vi "Test.vi"() -> ()   [LabVIEW 2010]
uses:
  <vilib>/DAQmx/read.llb/DAQmx Read.vi
  <vilib>/DAQmx/read.llb/DAQmx Read (Analog 2D DBL NChan NSamp).vi
  Create Dataset 2D Double.vi
  <vilib>/daqmx/miscellaneous.llb/DAQmx Fill In Error Info.vi
  Append To Dataset 2D Double.vi
  HDF5Tools.lvlib
panel:
  out "output array":dbl[](array[numeric])
  out "data 2":dbl[][](array[numeric]) format="%0.2f"
  out "size(s)":i32[](array[numeric])
  out "data":dbl[][](graph)
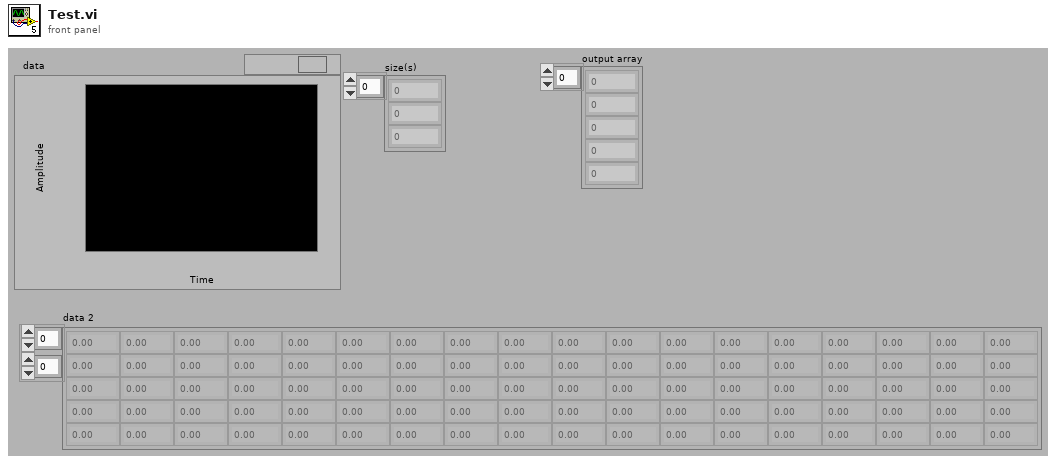
[diagram p1: front panel]
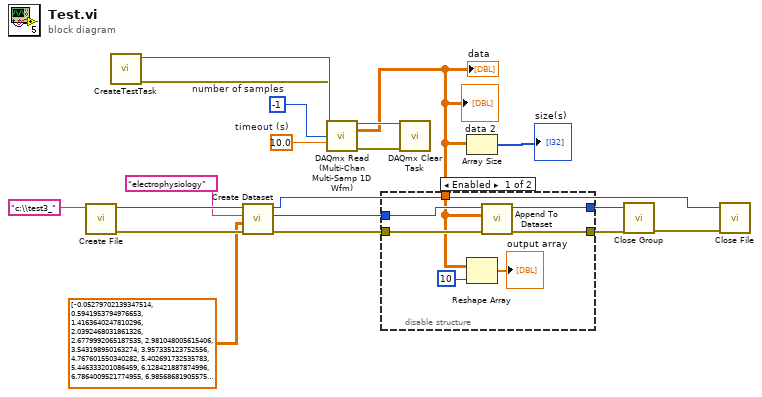
[diagram p0: block diagram]
diagram:
  w18 = 10.0  # timeout (s)
  w19 = -1  # number of samples
  n1 = call "Create File.vi"("File name"="c:\\test3_") -> ("Error out"=w9:errorcluster, "file_id"=w11:i32)  [unwired: 8 in]
  n2 = call "CreateTestTask.vi"() -> ("error out"=w14:errorcluster, "task out"=w15:refnum<k21>)  [unwired: 10 in]
  n3 = call-poly "Create Dataset.vi"("error in (no error)"=w9, "Data type"=dbl[][] [[-0.05279702139347514, 0.5941953794976653, 1.4163640247810296, 2.0392468031861326, 2.6779992065187535, 2.981048005615406, 3.543198950163274, 3.957335123752556, 4.767601550340282, 5.402691732535783, 5.446333201086459, 6.128421887874996, 6.7864009521774955, 6.985686819055758, 7.252723776970733, 7.696157719656972, 8.288827173680838, 8.26258125553148, 9.01364177373577, 8.951078829309976, 9.093600268562883, 9.45158238471633, 9.587694936979277, 9.609973448896756, 9.969481490524004, 9.938657795953246, 9.722586748863186, 9.497054963835566, 9.711600085451826, 9.554734946745201, 9.12961210974456, 9.220862453077793, 8.817712942899869, 8.655354472487563, 8.361461226233711, 7.8505813776055176, 7.7626880703146455, 6.990874965666677, 6.484572893459884, 5.98620563371685, 5.8729819635609, 4.979094821008942, 4.751731925412763, 4.029969176305429, 3.794366283150731, 3.174535355693228, 2.468947416608173, 1.6562395092623676, 1.1597033600878932, 0.5365153965880306, 0.06256294442579424, -0.32349620044557026, -0.9436323129978332, -1.9043549913022249, -2.652668843653676, -2.8943754387035736, -3.507797479171117, -3.9820551164281137, -4.6092104861598555, -5.171971800897244, -5.940122684408093, -6.327707754753257, -6.4226203192236095, -7.336954863124485, -7.196264534440138, -7.905209509567553, -7.9229102450636315, -8.770104068117313, -8.714255195776238, -8.944364757225257, -9.288308359019746, -9.182714316232795, -9.546189764091922, -9.67223120822779, -9.77782525101474, -9.749137852107303, -9.88952299569689, -9.640186773277993, -9.45890682699057, -9.431440168462172, -9.213538010803552, -8.856166264839626, -8.534501174962616, -8.512527848139896, -7.985168004394666, -7.706228827784051, -7.265541550950651, -7.314065981017487, -6.391796624652852, -6.2779625843073825, -5.897701956236458, -4.919278542435987, -4.865260780663473, -4.280831324198126, -3.3771782586138492, -3.293252357554857, -2.196722312082278, -1.564989165929136, -1.4697714163640248, -0.5999938962981048], [1.0998870815149389, 1.391338847010712, 2.226325266273995, 2.531510361033967, 3.3530686361278117, 3.595080416272469, 4.5603808709982605, 5.070039979247413, 5.275124362926115, 5.736564226203193, 6.082033753471481, 6.618549150059511, 7.011322367015595, 7.806329538865322, 7.701345866267891, 8.356578264717552, 8.833582567827387, 8.666646320993683, 8.846095156712547, 9.324320200201422, 9.720450453199867, 9.432355723746452, 9.642323068941312, 9.807123020111698, 9.539475692007203, 9.652699362163151, 9.492477187414167, 9.311807611316263, 9.423200170903653, 8.887295144505142, 8.654744102298043, 8.744163335062716, 8.549150059511094, 8.281197546311837, 7.417828913235877, 7.181920834986419, 6.910000915555284, 6.73818170720542, 5.87176122318186, 5.248878444776757, 5.085299233985412, 4.293954283272805, 3.6783959471419414, 3.083590197454756, 2.8113650929288614, 2.481460005493332, 1.6397595141453292, 0.7055879390850551, 0.5490279854731895, -0.10071108127079073, -0.9332560197759942, -1.6165654469435713, -1.9507431257057406, -2.621845149082919, -3.4580523087252417, -3.598437452314829, -4.082155827509385, -4.654683065279092, -5.513168736838892, -5.7777642139957885, -6.416821802423169, -7.009186071352275, -7.072969756157109, -7.345805230872524, -7.9396954252754295, -8.36634418774987, -8.741416669209876, -8.781395916623431, -9.282509842219307, -9.110385448774682, -9.584948271126438, -9.68230231635487, -9.35300759910886, -9.761345255897702, -9.761345255897702, -9.597460860011598, -9.765923032319101, -9.403057954649494, -9.547410504470962, -8.852198858607746, -9.069795831171605, -8.908658101138341, -8.37000640888699, -8.174382763145848, -7.771843623157445, -7.565843684194464, -6.823633533738212, -6.516006958220161, -6.160771507919553, -5.698416089358195, -5.094759971922971, -4.2780846583452865, -3.9252906888027588, -3.087252418591876, -2.5794244209112827, -2.325510422070986, -1.573839533677175, -0.9857478560747093, -0.5029450361644338, 0.195623645741142], [1.7447431867427594, 2.551347392193365, 3.0491042817468794, 3.7076937162388988, 3.783379619739372, 4.2695394756920075, 4.863734855189673, 5.7695242164372695, 6.2462233344523455, 6.539506210516678, 6.890774254585406, 7.264931180761131, 7.50144962920011, 7.911313211462752, 8.242744224372082, 8.625751518295846, 9.227271340067752, 9.216589861751151, 9.583422345652638, 9.604480117191077, 9.89410077211829, 9.45005645924253, 9.611499374370556, 9.957274086733603, 9.646900845362712, 9.44792016357921, 9.33622241889706, 9.519333475753044, 9.179357280190436, 8.966032898953214, 8.554948576311533, 8.285470137638479, 8.010193182164983, 7.353740043336283, 7.1254615924558244, 6.478469191564684, 6.355479598376415, 6.026184881130406, 5.041352580339976, 4.622943815424055, 4.001892147587512, 3.7336344492934965, 3.097933896908475, 2.412488174077578, 2.1713919492172002, 1.4307077242347483, 0.5606250190740685, -0.021362956633198035, -0.6103701895199438, -1.2573625904110843, -1.7676320688497573, -2.043519394512772, -3.0472731711783196, -3.5700552385021513, -3.8813440351573227, -4.850306711020234, -5.207983642078921, -5.344096194341868, -5.9071626941740165, -6.603900265511032, -7.260963774529252, -7.549363689077426, -8.038270210882901, -8.36512344737083, -8.207037568285164, -8.622699667348247, -9.266640217291787, -9.228797265541552, -9.411603137302775, -9.798577837458419, -9.714957121494185, -9.852595599230934, -9.738456373790704, -9.640186773277993, -9.368266853846858, -9.386577959532456, -9.67528305917539, -9.366130558183539, -9.199194311349833, -9.000518814661092, -8.860133671071505, -7.979674672688986, -8.092898342844935, -7.61040070802942, -7.206335642567217, -6.988738670003357, -6.370738853114414, -5.997497482222968, -5.424970244453261, -4.927823725089267, -4.5127719962157045, -3.728446302682577, -3.142796105838191, -2.6767784661397136, -1.8726157414471878, -1.4761803033539842, -0.619830927457503, -0.3793450727866451, 0.40406506546220283, 0.8655049287392804], [2.3856318857387007, 3.122653889584033, 3.7205114902188177, 4.082155827509385, 4.926297799615467, 5.007477034821619, 5.491805780205695, 6.428113650929289, 6.966154972991119, 6.853236487929929, 7.666859950560014, 7.71538438062685, 8.2586138492996, 8.788415173802912, 9.00967436750389, 9.079256569109164, 9.522385326700643, 9.599597155674918, 9.739371929074984, 9.605395672475357, 9.822992645039216, 9.517502365184484, 9.511703848384045, 9.712210455641346, 9.3496505630665, 9.391155735953856, 8.994109927671133, 9.12411877803888, 8.59431745353557, 8.665730765709403, 7.846919156468398, 7.849665822321238, 7.526169621875668, 6.9548631244850005, 6.290475173192541, 5.950804162724692, 5.361186559648427, 5.013580736716818, 4.878994109927671, 3.9179662465285197, 3.333536790063173, 2.707296975615711, 2.468947416608173, 1.8341624195074313, 0.8633686330759606, 0.5789361247596667, 0.18555253761406293, -0.8575701162755212, -1.076387829218421, -2.185735648670919, -2.409741508224738, -3.185827204199347, -3.795587023529771, -4.389477217932676, -4.555497909482101, -5.287942136906033, -5.720084231086154, -6.062501907406842, -6.923734244819483, -6.84408093508713, -7.425458540604877, -8.093203527939695, -8.25373088778344, -8.509475997192297, -8.873867000335704, -8.861659596545305, -9.185766167180395, -9.147007660145878, -9.642017883846552, -9.872127445295572, -9.491866817224647, -9.660023804437392, -9.753105258339183, -9.382915738395337, -9.503158665730766, -9.618823816644795, -9.302652058473464, -9.233069856868191, -8.537553025910215, -8.686178167058321, -8.088930936613055, -7.865840632343517, -7.526779992065188, -6.8422498245185706, -6.4308603167821285, -5.952330088198492, -5.634022034363841, -5.2052369762260815, -4.791405987731559, -4.214300973540452, -3.4751426740318, -2.652974028748436, -2.194280831324198, -1.8381298257393108, -0.9378337961973937, -0.2359080782494583, -0.044862208929715874, 0.9057893612475967, 1.402020325327311, 2.2019104586931975]] ("data 2"), "Dataset name"="electrophysiology", "loc_id"=w11) -> ("error out"=w7:errorcluster, "dataset_id"=w8:i32, "loc_id_out"=w2:i32)  [unwired: 5 in]
  n4 = call-poly "DAQmx Read (Multi-Chan Multi-Samp 1D Wfm).vi"("task/channels in"=w15, "number of samples per channel"=w19, "timeout"=w18, "error in"=w14) -> ("task out"=w16:refnum<k21>, "data"=w6:dbl[][], "error out"=w17:errorcluster)  [unwired: 9 in]
  "data" <- w6
  "data 2" <- w6
  n5 = disable-structure shown="Enabled" {
    disable-tunnel: w8 -> [w24 w27]
    disable-tunnel: w7 -> [w23 w28]
    disable-tunnel: w6 -> [w22 _]
    disable-tunnel: [w21 w27] -> w5
    disable-tunnel: [w20 w28] -> w4
    frame Enabled {
      n6 = Reshape Array(w22, 10 ("dimension size")) -> (→"output array":dbl[])
      n7 = call-poly "Append To Dataset.vi"("error in (no error)"=w23, "data"=w22, "dataset_id"=w24) -> ("error out"=w20:errorcluster, "dataset_out"=w21:i32)  [unwired: 7 in]
    }
    frame Disabled {
    }
  }
  n8 = call <vilib>:"DAQmx Clear Task.vi"("task in"=w16, "error in"=w17) -> ()  [unwired: 13 in, 1 out]
  n9 = Array Size(array=w6) -> (size(s)=→"size(s)":i32[])
  n10 = call "Close Group.vi"("error in (no error)"=w4, "group_id"=w5) -> ("error out"=w3:errorcluster)  [unwired: 9 in]
  n11 = call "Close File.vi"("error in (no error)"=w3, "file_id"=w2) -> ()  [unwired: 9 in, 1 out]
